vi "Change Lib Password.vi"(8 "error in (no error)":errorcluster, 10 "New Lib Password":string, 11 "Content in":T1) -> (0 "error out":errorcluster, 2 "Has Lib Password?":bool, 3 "Content out":T1)   [LabVIEW 2018, in "VI-Hacker.lvlib"]
uses:
  VI-Hacker.lvlib
  TypeDefs/Block.ctl
  TypeDefs/Content.ctl
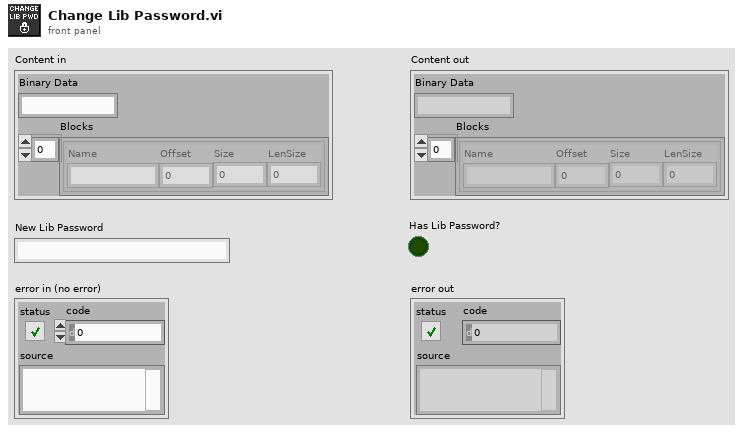
[diagram p1: front panel]
types:
  T1 = typedef "VI-Hacker.lvlib/Content.ctl" = cluster{"Binary Data":string, "Blocks":T2[]}
  T2 = typedef "VI-Hacker.lvlib/Block.ctl" = cluster{"Name":string, "Offset":i32, "Size":i32, "LenSize":i32}
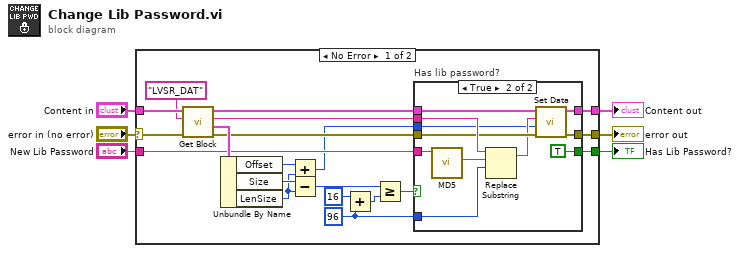
[diagram p0: block diagram]
diagram:
  n1 = case shown="No Error" "error in (no error)" {
    selector: "error in (no error)" -> [w26 w41]
    tunnel: "Content in" -> [w25 w40]
    tunnel: "New Lib Password" -> [w20 _]
    tunnel: [w15 w41] -> w3
    tunnel: [w14 w40] -> w2
    tunnel: [w7 _] -> w1
    frame No Error {
      w12 = 96 ("offset (0)")
      n2 = call "Get Block.vi"("error in (no error)"=w26, "Block Name"="LVSR_DAT", "Content in"=w25) -> ("error out"=w16:errorcluster, "Block out"=w23:T2, "Data out"=w19:string, "Content out"=w13:T1)  [unwired: 4 in, 1 out]
      n3 = Unbundle By Name(w23) -> ("Offset"=w11:i32, "Size"=w22:i32, "LenSize"=w10:i32)
      n4 = Add(x=w11, y=w10) -> (x+y=w8:i32)
      n5 = Subtract(x=w22, y=w10) -> (x-y=w21:i32)
      n6 = Add(x=16 ("y"), y=w12) -> (x+y=w17:i32)
      n7 = Greater Or Equal?(x=w21, y=w17) -> (x >= y?=w9:bool)
      n8 = case "Has lib password?" shown="True" w9 {
        tunnel: w20 -> [_ w39]
        tunnel: w19 -> [_ w38]
        tunnel: w16 -> [w27 w37]
        tunnel: [w27 w36] -> w15
        tunnel: [w28 w35] -> w14
        tunnel: w13 -> [w28 w34]
        tunnel: w12 -> [_ w33]
        tunnel: w8 -> [_ w30]
        tunnel: [_ TRUE] -> w7
        frame False {
        }
        frame True {
          n9 = call "MD5.vi"("Message String"=w39) -> ("MD5 (16-bytes)"=w31:string)  [unwired: 9 in, 1 out]
          n10 = Replace Substring(3:w33, 4:w31, 5:w38) -> (1:w32:string)  [unwired: 1 in, 1 out]
          n11 = call "Set Data.vi"("error in (no error)"=w37, "Offset"=w30, "Data in"=w32, "Content in"=w34) -> ("error out"=w36:errorcluster, "Content out"=w35:T1)  [unwired: 6 in]
        }
      }
    }
    frame Error {
    }
  }
  "error out" <- w3
  "Content out" <- w2
  "Has Lib Password?" <- w1
